vi "Set SR Cluster Item Visibility.vi"(10 "Screen Width":i16, 11 "SR List ref in":refnum<vi>) -> (0 "error out":errorcluster)   [LabVIEW 2018]
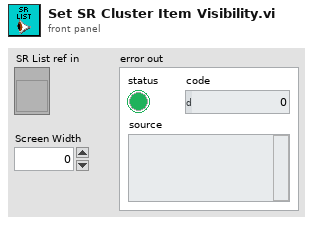
[diagram p1: front panel]
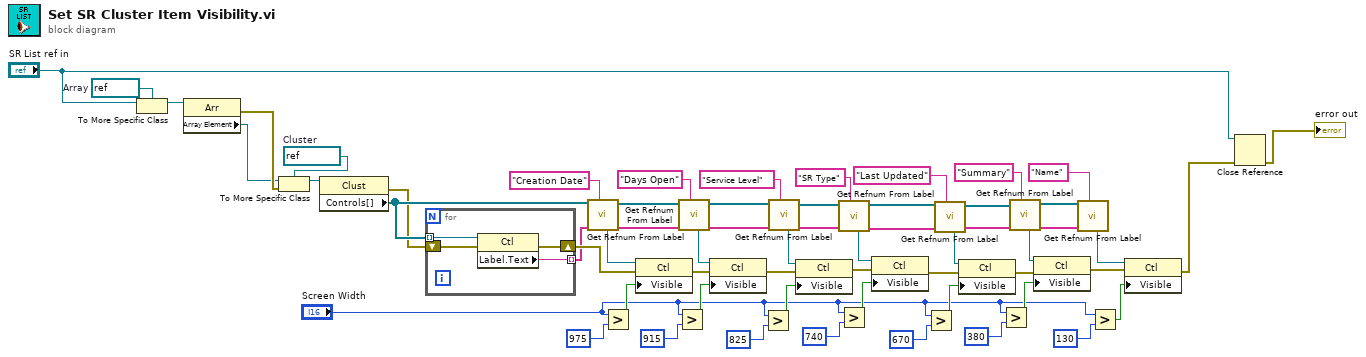
[diagram p0: block diagram]
diagram:
  w60 = refnum<vi> refnum  # Cluster
  w56 = refnum<vi> refnum  # Array
  n1 = To More Specific Class(target class=w56, reference="SR List ref in") -> (specific class reference=w57:refnum<vi>)  [unwired: 1 in, 1 out]
  n2 = property class="Arr"(reference=w57) -> (error out=w59:errorcluster, "Array Element"=w58:refnum<vi>)  [unwired: 1 in, 1 out]
  n3 = To More Specific Class(target class=w60, reference=w58, error in=w59) -> (specific class reference=w5:refnum<vi>)  [unwired: 1 out]
  n4 = property class="Clust"(reference=w5) -> (error out=w6:errorcluster, "Controls[]"=w8:refnum<vi>[])  [unwired: 1 in, 1 out]
  n5 = for {
    tunnel: w8 -> [w62] mode=indexing
    shift-right: [w63] -> w48
    shift-left: w6 -> [w64]
    tunnel: [w61] -> w7 mode=indexing
    n6 = property class="Ctl"(reference=w62, error in=w64) -> (error out=w63:errorcluster, "Label.Text"=w61:string)  [unwired: 1 out]
  }
  n7 = call "Get Refnum From Label.vi"("label"="Creation Date", "label array in"=w7, "controls[] in"=w8) -> ("label array out"=w12:string[], "controls[] out"=w11:refnum<vi>[], "refnum out"=w49:refnum<vi>)  [unwired: 6 in]
  n8 = Greater?(x="Screen Width", y=i16 975) -> (0:w44:bool)
  n9 = property class="Ctl"(reference=w49, error in=w48, "Visible"=w44) -> (error out=w45:errorcluster)  [unwired: 1 out]
  n10 = Greater?(x="Screen Width", y=i16 915) -> (0:w40:bool)
  n11 = call "Get Refnum From Label.vi"("label"="Days Open", "label array in"=w12, "controls[] in"=w11) -> ("label array out"=w15:string[], "controls[] out"=w14:refnum<vi>[], "refnum out"=w50:refnum<vi>)  [unwired: 6 in]
  n12 = property class="Ctl"(reference=w50, error in=w45, "Visible"=w40) -> (error out=w42:errorcluster)  [unwired: 1 out]
  n13 = Greater?(x="Screen Width", y=i16 825) -> (0:w39:bool)
  n14 = call "Get Refnum From Label.vi"("label"="Service Level", "label array in"=w15, "controls[] in"=w14) -> ("label array out"=w16:string[], "controls[] out"=w17:refnum<vi>[], "refnum out"=w51:refnum<vi>)  [unwired: 6 in]
  n15 = property class="Ctl"(reference=w51, error in=w42, "Visible"=w39) -> (error out=w47:errorcluster)  [unwired: 1 out]
  n16 = call "Get Refnum From Label.vi"("label"="SR Type", "label array in"=w16, "controls[] in"=w17) -> ("label array out"=w20:string[], "controls[] out"=w19:refnum<vi>[], "refnum out"=w52:refnum<vi>)  [unwired: 6 in]
  n17 = Greater?(x="Screen Width", y=i16 740) -> (0:w36:bool)
  n18 = property class="Ctl"(reference=w52, error in=w47, "Visible"=w36) -> (error out=w46:errorcluster)  [unwired: 1 out]
  n19 = Greater?(x="Screen Width", y=i16 670) -> (0:w34:bool)
  n20 = call "Get Refnum From Label.vi"("label"="Last Updated", "label array in"=w20, "controls[] in"=w19) -> ("label array out"=w24:string[], "controls[] out"=w23:refnum<vi>[], "refnum out"=w53:refnum<vi>)  [unwired: 6 in]
  n21 = property class="Ctl"(reference=w53, error in=w46, "Visible"=w34) -> (error out=w35:errorcluster)  [unwired: 1 out]
  n22 = Greater?(x="Screen Width", y=i16 380) -> (0:w30:bool)
  n23 = call "Get Refnum From Label.vi"("label"="Summary", "label array in"=w24, "controls[] in"=w23) -> ("label array out"=w26:string[], "controls[] out"=w25:refnum<vi>[], "refnum out"=w32:refnum<vi>)  [unwired: 6 in]
  n24 = property class="Ctl"(reference=w32, error in=w35, "Visible"=w30) -> (error out=w54:errorcluster)  [unwired: 1 out]
  n25 = call "Get Refnum From Label.vi"("label"="Name", "label array in"=w26, "controls[] in"=w25) -> ("refnum out"=w55:refnum<vi>)  [unwired: 6 in, 2 out]
  n26 = Greater?(x="Screen Width", y=i16 130) -> (0:w29:bool)
  n27 = property class="Ctl"(reference=w55, error in=w54, "Visible"=w29) -> (error out=w3:errorcluster)  [unwired: 1 out]
  n28 = Close Reference(reference="SR List ref in", error in (no error)=w3) -> (error out=→"error out":errorcluster)
